vi "S2DS_Export Channel names (SubVI).vi"(8 "error in (no error)":errorcluster, 11 "All channel info (in)":T1={"WCl names with units"=[], "RC  names with units"=[], "DC  names with units"=[""], "AC names with units"=[], "Indicator captions"=[], "Graph channels"=[], "Channel numbers"=[], "User info"=""}) -> (0 "error out":errorcluster)   [LabVIEW 2025]
uses:
  TYPE DEFS/S2DS_Display info.ctl
  <vilib>/Utility/sysdir.llb/System Directory Type.ctl
  <vilib>/Utility/config.llb/Write Key (String).vi
  <vilib>/Utility/config.llb/NI_LVConfig.lvlib
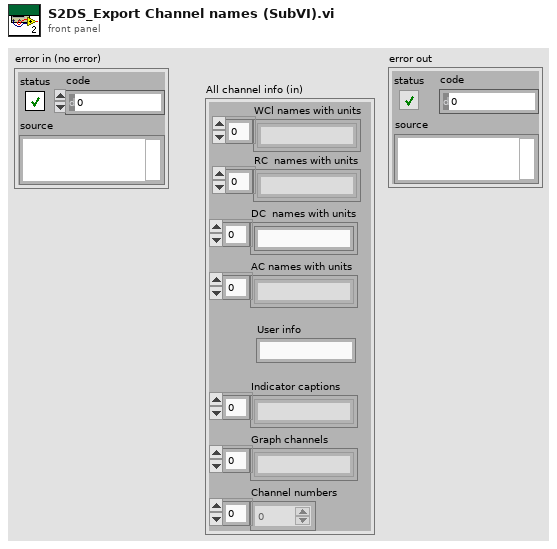
[diagram p1: front panel]
types:
  T1 = typedef "S2DS_Display info.ctl" = cluster{"WCl names with units":string[], "RC  names with units":string[], "DC  names with units":string[], "AC names with units":string[], "Indicator captions":string[], "Graph channels":string[], "Channel numbers":i32[], "User info":string}
  T2 = typedef "System Directory Type.ctl" = i32
  T3 = typedef "NI_LVConfig.lvlib/Config Data RefNum.ctl" = refnum<k1>
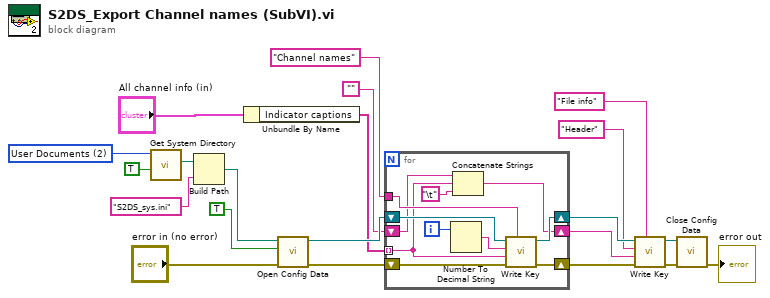
[diagram p0: block diagram]
diagram:
  w21 = T2 2 items=["User Home"=0, "User Desktop"=1, "User Documents"=2, "User Application Data"=3, "User Preferences"=4, "User Temporary"=5, "Public Documents"=6, "Public Application Data"=7, "Public Preferences"=8, "Public Cache"=13, "System Core Libraries"=9, "System Installed Libraries"=10, "Application Files"=11, "Boot Volume Root"=12] ("system directory type")
  n1 = call <vilib>:"Get System Directory.vi"("create directory if not found? (F)"=TRUE, "system directory type"=w21) -> ("system directory"=w19:path)  [unwired: 9 in]
  n2 = Build Path(base path=w19, name or relative path="S2DS_sys.ini") -> (appended path=w17:path)
  n3 = Unbundle By Name("All channel info (in)") -> ("Indicator captions"=w1:string[])
  n4 = call <vilib>:"Open Config Data.vi"("error in (no error)"="error in (no error)", "create file if necessary (T)"=TRUE, "configuration file path"=w17) -> ("error out"=w15:errorcluster, "refnum"=w14:T3)  [unwired: 6 in, 1 out]
  n5 = for {
    shift-right: [w30] -> w8
    shift-left: w15 -> [w31]
    shift-right: [w29] -> w9
    shift-left: w14 -> [w32]
    tunnel: w1 -> [w25] mode=indexing
    tunnel: "Channel names" -> [w26]
    shift-right: [w24] -> w5
    shift-left: "" -> [w23]
    i -> [w28]
    n6 = Number To Decimal String(number=w28) -> (decimal integer string=w27:string)  [unwired: 1 in]
    n7 = Concatenate Strings(w23, w25, "\t") -> (w24:string)
    n8 = call-poly <vilib>:"Write Key.vi"("section"=w26, "error in (no error)"=w31, "value"=w25, "key"=w27, "refnum"=w32) -> ("error out"=w30:errorcluster, "refnum out"=w29:T3)  [unwired: 4 in, 1 out]
  }
  n9 = call-poly <vilib>:"Write Key.vi"("section"="File info", "error in (no error)"=w8, "value"=w5, "key"="Header", "refnum"=w9) -> ("error out"=w6:errorcluster, "refnum out"=w7:T3)  [unwired: 4 in, 1 out]
  n10 = call <vilib>:"Close Config Data.vi"("error in (no error)"=w6, "refnum"=w7) -> ("error out"=→"error out":errorcluster)  [unwired: 8 in, 1 out]
